vi "Read from DB.vi"() -> ()   [LabVIEW 2017]
uses:
  Type Definitions/DB Record.ctl
panel:
  out "DB Record":T1 {"Balance" format="%.2f"; "Account" format="%05d"}
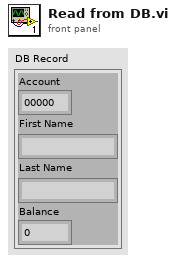
[diagram p1: front panel]
types:
  T1 = typedef "DB Record.ctl" = cluster{"Account":i32, "First Name":string, "Last Name":string, "Balance":fxp<+/-,64,35>}
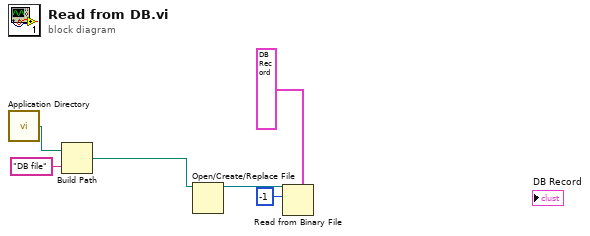
[diagram p0: block diagram]
diagram:
  n1 = call <vilib>:"Application Directory.vi"() -> ("Application Directory"=w6:path)
  n2 = Build Path(base path=w6, name or relative path="DB file") -> (appended path=w4:path)
  n3 = Open/Create/Replace File(file path (use dialog)=w4) -> (refnum out=w3:refnum<file>)  [unwired: 5 in, 2 out]
  n4 = Read from Binary File(5:T1 {"Account"=0, "First Name"="", "Last Name"="", "Balance"=0.0} ("DB Record"), 10:-1 ("count (1)"), 11:w3) -> ()  [unwired: 3 in, 4 out]
